vi "Pointer_Add or Replace.vi"(8 "Error":errorcluster, 9 "Pointer":refnum<class "_Pointer.lvclass">, 10 "Index":i32=-1, 11 "WavBuf":refnum<class "WavBuf.lvclass">) -> (0 "Error Out":errorcluster, 1 "Pointer Out":refnum<class "_Pointer.lvclass">, 3 "WavBuf Out":refnum<class "WavBuf.lvclass">)   [LabVIEW 2024, in "WavBuf.lvclass"]
uses:
  WavBuf.lvclass
  Pointer/_Pointer.lvclass
  WavBuf.lvclass/WavBuf.ctl
panel:
  out "Index Out":i32
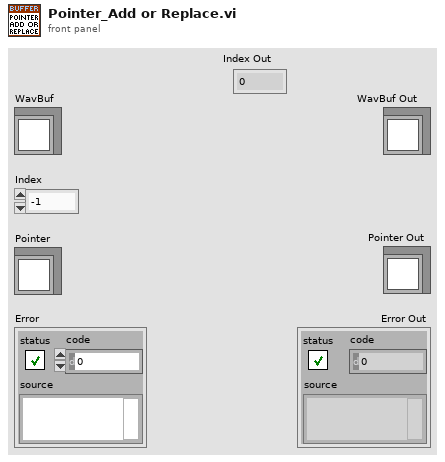
[diagram p1: front panel]
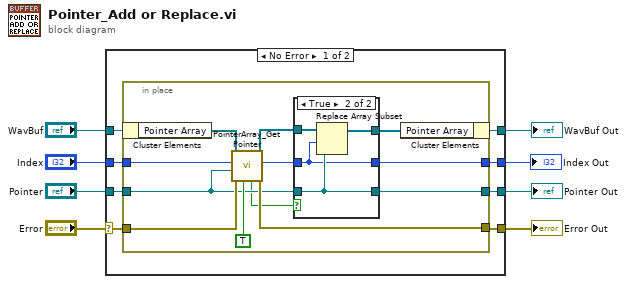
[diagram p0: block diagram]
diagram:
  n1 = case shown="No Error" "Error" {
    selector: "Error" -> [w12 w39]
    tunnel: [w11 w39] -> w8
    tunnel: [w15 w38] -> w7
    tunnel: "WavBuf" -> [w16 w38]
    tunnel: "Index" -> [w14 w36]
    tunnel: "Pointer" -> [w13 w37]
    tunnel: [w10 w37] -> w2
    tunnel: [w9 w36] -> w1
    frame No Error {
      n2 = in-place {
        in-place-border: w14 -> [w27]
        in-place-border: w13 -> [w20]
        in-place-border: w12 -> [w23]
        in-place-border: [w22] -> w11
        in-place-border: [w19] -> w10
        in-place-border: [w18] -> w9
        n3 = in-place-cluster #1(w16) -> ("Pointer Array"=w28:refnum<class "_Pointer.lvclass">[])
        n4 = call "PointerArray_Get Pointer.vi"("Create If Not Found"=TRUE, "Error"=w23, "Pointer"=w20, "Index"=w27, "Pointer Array"=w28) -> ("Error Out"=w22:errorcluster, "Index Out"=w21:i32, "Pointer Array Out"=w25:refnum<class "_Pointer.lvclass">[], "Found Out"=w17:bool)  [unwired: 2 in, 1 out]
        n5 = case shown="True" w17 {
          tunnel: w25 -> [w31 w35]
          tunnel: [w31 w34] -> w24
          tunnel: w21 -> [w29 w32]
          tunnel: w20 -> [w30 w33]
          tunnel: [w30 w33] -> w19
          tunnel: [w29 w32] -> w18
          frame False {
          }
          frame True {
            n6 = Replace Array Subset(array=w35, new element=w33, index=w32) -> (w34:refnum<class "_Pointer.lvclass">[])
          }
        }
        n7 = in-place-cluster #1("Pointer Array"=w24) -> (w15:refnum<class "WavBuf.lvclass">)
      }
    }
    frame Error {
    }
  }
  "Error Out" <- w8
  "WavBuf Out" <- w7
  "Pointer Out" <- w2
  "Index Out" <- w1
